vi "OE1022D_GPIB_Query Data.vi"(0 "VISA resource name":refnum<visa-resource-name>, 9 "Timeout":u32=1000, 11 "Error in (no error)":errorcluster caption="error out（no error）") -> (4 "VISA resource  out":refnum<visa-resource-name>, 6 "Parameter Values":T1, 8 "Data Array":dbl[](array[numeric]), 10 "Output String":string, 15 "Error out":errorcluster caption="error out")   [LabVIEW 2011]
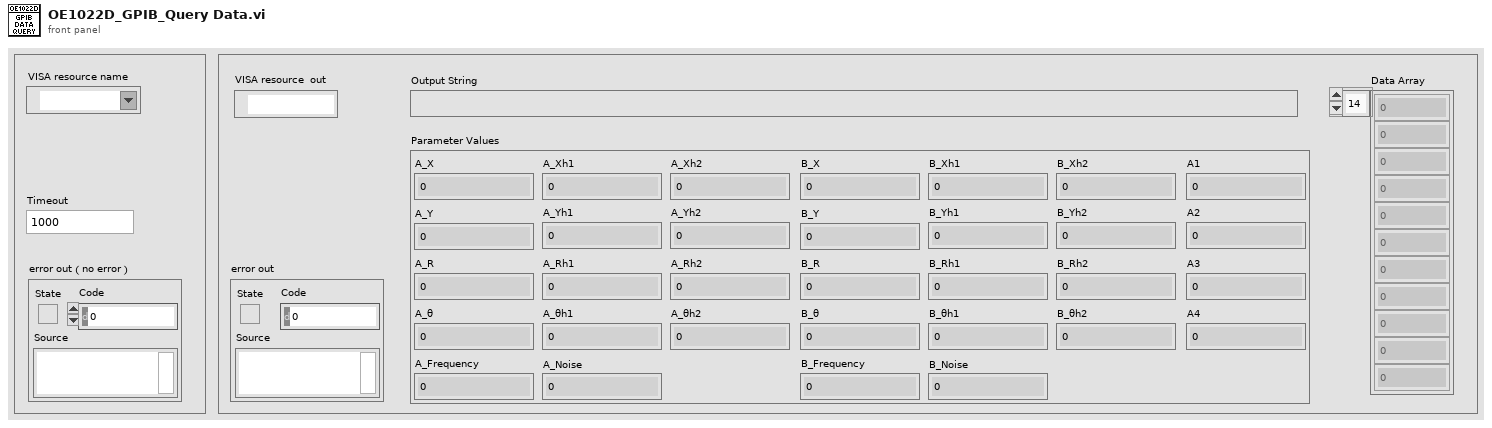
[diagram p1: front panel]
types:
  T1 = cluster{"A_X":dbl, "A_Y":dbl, "A_R":dbl, "A_θ":dbl, "A_Frequency":dbl, "A_Noise":dbl, "A_Xh1":dbl, "A_Yh1":dbl, "A_Rh1":dbl, "A_θh1":dbl, "A_Xh2":dbl, "A_Yh2":dbl, "A_Rh2":dbl, "A_θh2":dbl, "B_X":dbl, "B_Y":dbl, "B_R":dbl, "B_θ":dbl, "B_Frequency":dbl, "B_Noise":dbl, "B_Xh1":dbl, "B_Yh1":dbl, "B_Rh1":dbl, "B_θh1":dbl, "B_Xh2":dbl, "B_Yh2":dbl, "B_Rh2":dbl, "B_θh2":dbl, "A1":dbl, "A2":dbl, "A3":dbl, "A4":dbl}
  T2 = enum16{"ISRC", "IGND", "ICPL", "ILIN", "PHAS", "FMOD", "RSLP", "FREQ", "SWPT", "SLLM", "SULM", "SSLL", "SSLG", "STLM", "SWRM", "IRNG", "SENS", "RMOD", "OFLT", "OFSL", "SYNC", "DMOD", "HARM", "DARB", "SWVT", "SLVL", "SVLL", "SVUL", "SVSL", "SVSG", "SVTM", "SVRM", "RALL", "SNAP", "OUTP", "OAUX", "COUT", "CAUX", "COFP", "CEXP", "FPOP", "OEXP", "*IDN", "*RST", "OVLD", "INOV", "GNOV", "*PLL", "SSET", "RSET", "AGAN", "APHS", "ARSV", "ASCL", "EQCD", "EQCS", "SPED", "SRAT", "SLEN", "SSLE", "STRG", "SPRM", "STRD", "PAUS", "REST", "SPTS", "TRCA", "TEMP", "RSTU", "IHNZ", "DEQU", "SADD", "ARNG", "CSPE", "ISRCD", "IGNDD", "ICPLD", "ILIND", "PHASD", "FMODD", "RSLPD", "FREQD", "SWPTD", "SLLMD", "SULMD", "SSLLD", "SSLGD", "STLMD", "SWRMD", "SENSD", "RMODD", "OFLTD", "OFSLD", "SYNCD", "HARMD", "EQCDD", "EQCSD", "SNAPD", "OUTPD", "SWVTD", "SLVLD", "SVLLD", "SVULD", "SVSLD", "SVSGD", "SVTMD", "SVRMD", "SVDCD", "ARSVD", "AGAND", "APHSD", "ASCLD", "FPOPD", "CAUXD", "OEXPD", "SPEDD", "SRATD", "SLEND", "SSLED", "STRGD", "SPRMD", "STRDD", "PAUSD", "RESTD", "SPTSD", "TRCAD", "*IDND", "*RSTD", "INOVD", "GNOVD", "*PLLD", "SSETD", "RSETD", "RALLD"}
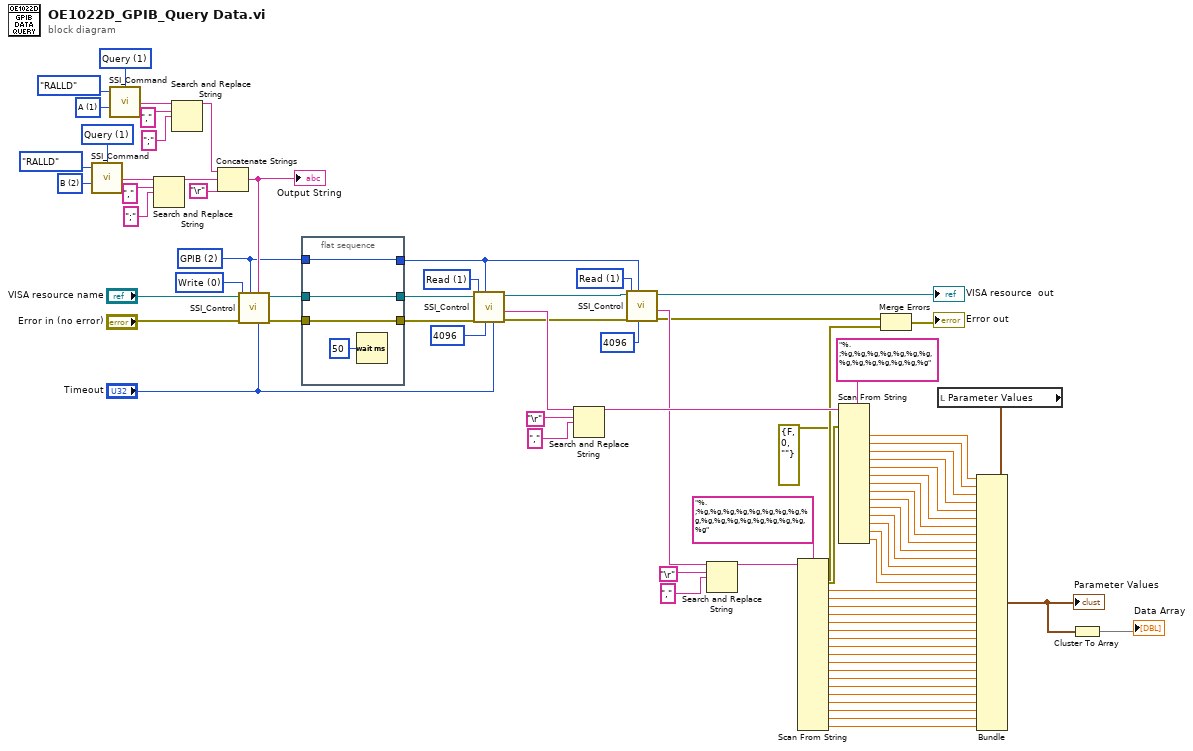
[diagram p0: block diagram]
diagram:
  w48 = u16 1 items=["Write", "Read"] ("Control")
  w59 = u16 1 items=["A"=1, "B"=2] ("channel")
  w55 = u16 1 items=["Set", "Query"] ("Opera")
  w60 = u16 2 items=["A"=1, "B"=2] ("channel")
  w71 = u16 1 items=["Set", "Query"] ("Opera")
  w73 = u16 2 items=["USB", "RS232", "GPIB", "Ethernet"] ("Remote Mode")
  w76 = u16 1 items=["Write", "Read"] ("Control")
  w81 = u16 0 items=["Write", "Read"] ("Control")
  n1 = call "SSI_Command.vi"("Opera"=w71, "channel"=w60, "Command Type"=T2."RALLD") -> ("Output string"=w70:string)  [unwired: 1 in]
  n2 = call "SSI_Command.vi"("Opera"=w55, "channel"=w59, "Command Type"=T2."RALLD") -> ("Output string"=w56:string)  [unwired: 1 in]
  n3 = Search and Replace String(input string=w70, search string="," ("搜索字符串"), replace string=";") -> (result string=w66:string)  [unwired: 5 in, 3 out]
  n4 = Search and Replace String(input string=w56, search string="," ("搜索字符串"), replace string=";") -> (result string=w53:string)  [unwired: 5 in, 3 out]
  n5 = Concatenate Strings(w53, w66, "\r") -> (w74:string)
  "Output String" <- w74
  n6 = call "SSI_Control.vi"("Tineout"="Timeout", "Write Buffer"=w74, "Remote Mode"=w73, "Error in (no error)"="Error in (no error)", "Control"=w81, "VISA resource name"="VISA resource name") -> ("Error out"=w79:errorcluster, "VISA resource  out"=w80:refnum<visa-resource-name>)  [unwired: 2 in, 2 out]
  n7 = flat-sequence {
    tunnel: w80 -> [w87]
    tunnel: w79 -> [w86]
    tunnel: [w87] -> w78
    tunnel: [w86] -> w77
    tunnel: [w84] -> w27
    tunnel: w73 -> [w84]
    frame #0 {
      n8 = Wait (ms)(milliseconds to wait=u32 50 ("等待时间（毫秒）")) -> ()  [unwired: 1 out]
    }
  }
  n9 = call "SSI_Control.vi"("Tineout"="Timeout", "Number of bytes"=u32 4096, "Remote Mode"=w27, "Error in (no error)"=w77, "Control"=w76, "VISA resource name"=w78) -> ("Error out"=w6:errorcluster, "Read Buffer"=w63:string, "VISA resource  out"=w26:refnum<visa-resource-name>)  [unwired: 2 in, 1 out]
  n10 = Search and Replace String(input string=w63, search string="\r", replace string=",") -> (result string=w62:string)  [unwired: 5 in, 3 out]
  n11 = call "SSI_Control.vi"("Number of bytes"=u32 4096, "Remote Mode"=w27, "Error in (no error)"=w6, "Control"=w48, "VISA resource name"=w26) -> ("Error out"=w4:errorcluster, "Read Buffer"=w52:string, "VISA resource  out"=→"VISA resource  out":refnum<visa-resource-name>)  [unwired: 3 in, 1 out]
  n12 = Search and Replace String(input string=w52, search string="\r", replace string=",") -> (result string=w28:string)  [unwired: 5 in, 3 out]
  n13 = Scan From String(format string="%.;%g,%g,%g,%g,%g,%g,%g,%g,%g,%g,%g,%g,%g,%g" ("格式字符串"), input string=w62, error in=errorcluster {"status"=FALSE, "code"=0, "source"=""} ("error constant")) -> (error out=w3:errorcluster, output 1=w11:dbl, output 2=w10:dbl, output 3=w13:dbl, output 4=w14:dbl, output 5=w15:dbl, output 6=w16:dbl, output 7=w17:dbl, output 8=w18:dbl, output 9=w19:dbl, output 10=w20:dbl, output 11=w21:dbl, output 12=w22:dbl, output 13=w23:dbl, output 14=w24:dbl)  [unwired: 15 in, 2 out]
  n14 = Scan From String(format string="%.;%g,%g,%g,%g,%g,%g,%g,%g,%g,%g,%g,%g,%g,%g,%g,%g,%g,%g" ("格式字符串"), input string=w28, error in=w3) -> (error out=w2:errorcluster, output 1=w29:dbl, output 2=w30:dbl, output 3=w31:dbl, output 4=w32:dbl, output 5=w33:dbl, output 6=w34:dbl, output 7=w35:dbl, output 8=w36:dbl, output 9=w37:dbl, output 10=w38:dbl, output 11=w39:dbl, output 12=w40:dbl, output 13=w41:dbl, output 14=w42:dbl, output 15=w43:dbl, output 16=w44:dbl, output 17=w45:dbl, output 18=w46:dbl)  [unwired: 19 in, 2 out]
  n15 = Merge Errors(w4, w2) -> (→"Error out":errorcluster)
  n16 = local read "Parameter Values"() -> (w12:T1)
  n17 = Bundle(cluster=w12, "A_X"=w11, "A_Y"=w10, "A_R"=w13, "A_θ"=w14, "A_Frequency"=w15, "A_Noise"=w16, "A_Xh1"=w17, "A_Yh1"=w18, "A_Rh1"=w19, "A_θh1"=w20, "A_Xh2"=w21, "A_Yh2"=w22, "A_Rh2"=w23, "A_θh2"=w24, "B_X"=w29, "B_Y"=w30, "B_R"=w31, "B_θ"=w32, "B_Frequency"=w33, "B_Noise"=w34, "B_Xh1"=w35, "B_Yh1"=w36, "B_Rh1"=w37, "B_θh1"=w38, "B_Xh2"=w39, "B_Yh2"=w40, "B_Rh2"=w41, "B_θh2"=w42, "A1"=w43, "A2"=w44, "A3"=w45, "A4"=w46) -> (w8:T1)
  "Parameter Values" <- w8
  n18 = Cluster To Array(cluster=w8) -> (array=→"Data Array":dbl[])
